vi "To 1D String Tree Data.vi"(10 "1D String":string[](array[string])) -> (3 "1D String Tree Data":refnum<class "1D String.lvclass">)   [LabVIEW 2020, in "NI_VIAnCFGDataStructure.lvlib" / "1D String.lvclass"]
doc: "Convert a 1D String value to Tree Data type."
uses:
  <vilib>/addons/analyzer/VIAnCFGDataStructure/Data Types/String Array/1D String.lvclass
  <vilib>/addons/analyzer/VIAnCFGDataStructure/Data Types/String Array/1D String.lvclass/1D String.ctl
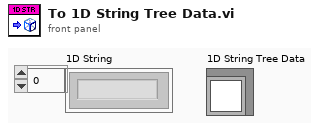
[diagram p1: front panel]
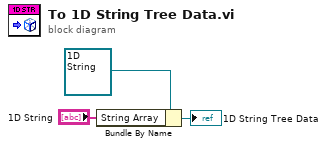
[diagram p0: block diagram]
diagram:
  n1 = Bundle By Name(cluster=refnum<class "1D String.lvclass"> refnum ("StringArray.lvclass"), "String Array"="1D String") -> (→"1D String Tree Data":refnum<class "1D String.lvclass">)
